vi "Write Device IDs.vi"(8 "error in":errorcluster, 9 "Microgrid ID":u8=1 min=1 max=232 step=1, 10 "Device ID Array":T1[](array[typedef]), 11 "EMS Generic in":refnum<class "EMS Generic.lvclass">) -> (0 "error out":errorcluster, 3 "dup EMS Generic out":refnum<class "EMS Generic.lvclass">)   [LabVIEW 2018, in "EMS Generic Actor.lvlib" / "EMS Generic.lvclass"]
uses:
  EMS Generic.lvclass
  <vilib>/ORNL/CSEISMIC DDS/CSEISMIC DDS Base/Data Types/Controls/DeviceID.ctl
  EMS Generic.lvclass/EMS Generic.ctl
  <vilib>/ORNL/CSEISMIC DDS/CSEISMIC DDS Base/CSEISMIC DDS.lvclass
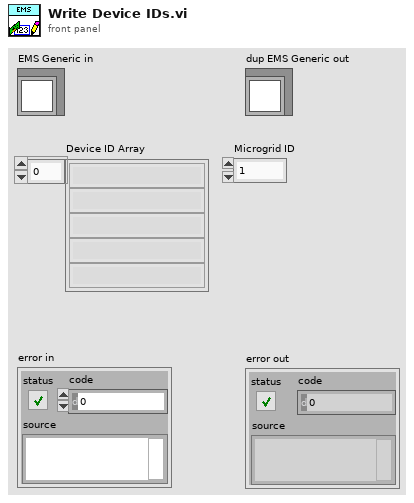
[diagram p1: front panel]
types:
  T1 = typedef "CSEISMIC DDS.lvlib/CSEISMIC DDS.lvclass/DeviceID.ctl" = string
  T2 = typedef "EMS Generic Actor.lvlib/EMS Generic.lvclass/Global Configuration.ctl" = cluster{"Microgrid ID":u8, "VF Device ID":T1, "Ongrid VF Priority":T1[], "Offgrid VF Priority":T1[], "AutoSwap Offgrid VF":u32, "AutoSwap Offgrid VF Delay (sec)":dbl, "AutoSwap Resynch VF":u32, "PCC Device ID":T1, "Device ID Array":T1[], "Nominal Voltage":dbl, "Nominal Frequency":dbl, "Resynch Timeout (sec)":dbl, "Island VF Activate Timeout (sec)":dbl, "Island PCC Target Power (kW)":dbl, "Island PCC Target Power Timeout (sec)":dbl, "Island Grid Settle Time (sec)":dbl, "Island PCC Failure Timeout (sec)":dbl, "Activation Devices Present Timeout (sec)":dbl, "Activation Devices Activated Timeout (sec)":dbl, "Blackstart VF GenMode Wait (sec)":dbl, "Blackstart VF DERCtrl Wait (sec)":dbl, "Blackstart Success Wait (sec)":dbl, "OnGrid Optimization Delay (sec)":dbl, "OffGrid Optimization Delay (sec)":dbl, "Resynch Frequency (Hz)":dbl, "Optimization Path":string}
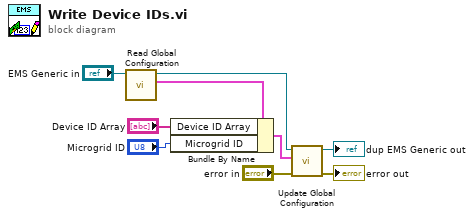
[diagram p0: block diagram]
diagram:
  n1 = call "Read Global Configuration.vi"("EMS Generic in"="EMS Generic in") -> ("Global Configuration"=w7:T2, "dup EMS Generic out"=w9:refnum<class "EMS Generic.lvclass">)  [unwired: 8 in, 1 out]
  n2 = Bundle By Name(cluster=w7, "Device ID Array"="Device ID Array", "Microgrid ID"="Microgrid ID") -> (w8:T2)
  n3 = call "Update Global Configuration.vi"("error in (no error)"="error in", "Global Configuration"=w8, "EMS Generic in"=w9) -> ("error out"=→"error out":errorcluster, "EMS Generic out"=→"dup EMS Generic out":refnum<class "EMS Generic.lvclass">)  [unwired: 7 in]
